vi "用文件函数读取前面板记录数据.vi"() -> ()   [LabVIEW 2010]
panel:
  out "记录":T1
  out "波形":dbl[](graph)
  in  "文件路径":path
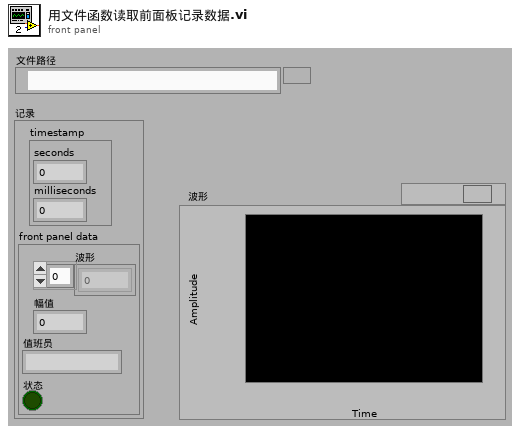
[diagram p1: front panel]
types:
  T1 = cluster{"timestamp":cluster{"seconds":u32, "milliseconds":u16}, "front panel data":cluster{"波形":dbl[], "幅值":dbl, "值班员":string, "状态":bool}}
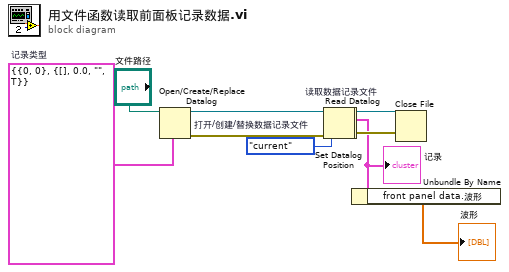
[diagram p0: block diagram]
diagram:
  w6 = T1 {"timestamp"={"seconds"=0, "milliseconds"=0}, "front panel data"={"波形"=[], "幅值"=0.0, "值班员"="", "状态"=TRUE}}  # 记录类型
  n1 = Open/Create/Replace Datalog "打开/创建/替换数据记录文件"(5:w6, 11:"文件路径") -> (0:w9:errorcluster, 3:w10:refnum<k1>)  [unwired: 4 in, 1 out]
  n2 = Set Datalog Position(4:w9, 5:enum16{"start", "end", "current"}."current" ("自（0:起始）"), 7:w10) -> (0:w2:errorcluster, 3:w3:refnum<k1>)  [unwired: 1 in]
  n3 = Read Datalog "读取数据记录文件"(4:w2, 7:w3) -> (0:w7:errorcluster, 2:w5:T1, 3:w8:refnum<k1>)  [unwired: 1 in]
  "记录" <- w5
  n4 = Unbundle By Name(w5) -> ("front panel data.波形"=→"波形":dbl[])
  n5 = Close File(refnum=w8, error in=w7) -> ()  [unwired: 2 out]
